vi "Start AsyncSum LowLevel.vi"(7 "LVUserEventCallBackRef":refnum<user-event>, 8 "error in":errorcluster, 9 "B":i32, 10 "A":i32, 11 "path in":path) -> (0 "error out":errorcluster, 2 "Handle":u64, 3 "dup path":path)   [LabVIEW 2016, in "DemoSkeleton.lvlib"]
uses:
  DemoSkeleton.lvlib
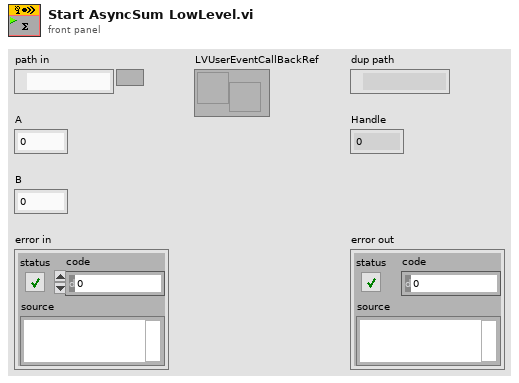
[diagram p1: front panel]
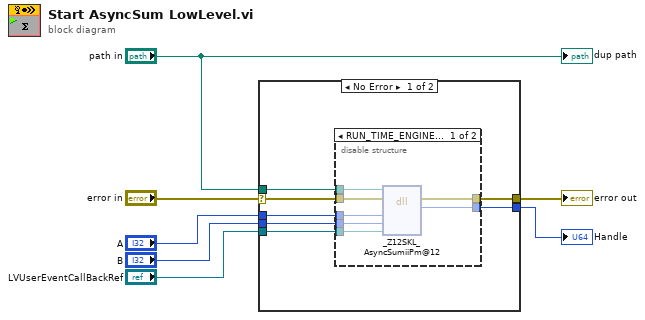
[diagram p0: block diagram]
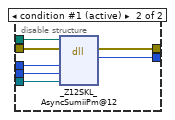
[diagram p2: hidden frame]
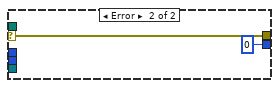
[diagram p3: hidden frame]
diagram:
  n1 = case shown="No Error" "error in" {
    selector: "error in" -> [w14 w30]
    tunnel: [w13 w30] -> w6
    tunnel: "A" -> [w12 _]
    tunnel: "B" -> [w11 _]
    tunnel: "LVUserEventCallBackRef" -> [w10 _]
    tunnel: [w9 u64 0 ("Handle")] -> w2
    tunnel: "path in" -> [w8 _]
    frame No Error {
      n2 = disable-structure shown="RUN_TIME_ENGINE==True" {
        disable-tunnel: [w18 w25] -> w9
        disable-tunnel: w14 -> [w21 w28]
        disable-tunnel: [w19 w26] -> w13
        disable-tunnel: w10 -> [w20 w27]
        disable-tunnel: w12 -> [w17 w24]
        disable-tunnel: w11 -> [w16 w23]
        disable-tunnel: w8 -> [w15 w22]
        frame condition #0 {
          n3 = dll-call lib="C:/Users/loic.wohleber/Desktop/PostLVUserEvent_Demo/Sources/LabVIEW/Library/DemoSkeleton/skeleton_lv_event_lvrt.dll" fn="_Z12SKL_AsyncSumiiPm@12" label="AsyncSum_RT"(path in=w15, error in=w21, "A"=w17, "B"=w16, "CallBackRefEvent"=w20) -> (error out=w19:errorcluster, "Handle"=w18:u64)  [unwired: 4 in, 1 out]
        }
        frame condition #1 (active) {
          n4 = dll-call lib="C:/Users/loic.wohleber/Desktop/PostLVUserEvent_Demo/Sources/LabVIEW/Library/DemoSkeleton/skeleton_lv_event_lv.dll" fn="_Z12SKL_AsyncSumiiPm@12" label="AsyncSum"(path in=w22, error in=w28, "A"=w24, "B"=w23, "CallBackRefEvent"=w27) -> (error out=w26:errorcluster, "Handle"=w25:u64)  [unwired: 4 in, 1 out]
        }
      }
    }
    frame Error {
    }
  }
  "error out" <- w6
  "Handle" <- w2
  "dup path" <- "path in"
